vi "Set Next Empty Row.vi"(8 "error in (no error)":errorcluster, 10 "Next Empty Row":i32, 11 "Excel Sheet in":refnum<class "Excel Sheet.lvclass">) -> (0 "error out":errorcluster, 3 "Excel Sheet out":refnum<class "Excel Sheet.lvclass">)   [LabVIEW 2016, in "Excel Sheet.lvclass"]
uses:
  Excel Sheet.lvclass
  Excel Sheet.lvclass/Excel Sheet.ctl
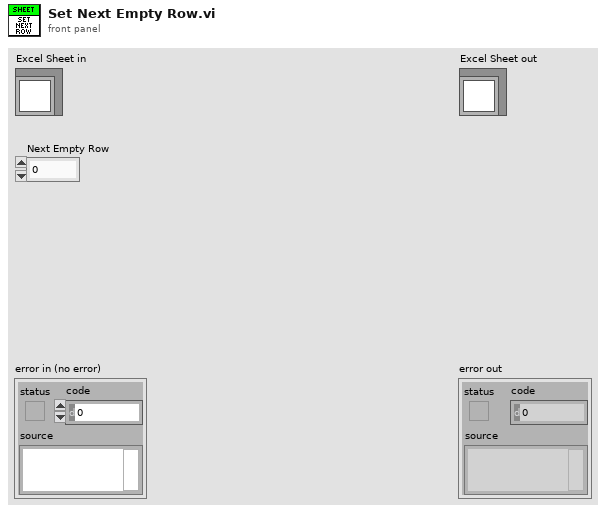
[diagram p1: front panel]
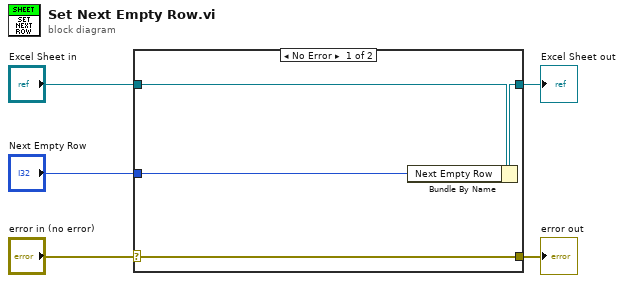
[diagram p0: block diagram]
diagram:
  n1 = case shown="No Error" "error in (no error)" {
    selector: "error in (no error)" -> [w9 w10]
    tunnel: [w9 w10] -> w4
    tunnel: [w7 w11] -> w2
    tunnel: "Excel Sheet in" -> [w8 w11]
    tunnel: "Next Empty Row" -> [w6 _]
    frame No Error {
      n2 = Bundle By Name(cluster=w8, "Next Empty Row"=w6) -> (w7:refnum<class "Excel Sheet.lvclass">)
    }
    frame Error {
    }
  }
  "error out" <- w4
  "Excel Sheet out" <- w2
